vi "Move Impl.vi"(6 "Mode":enum16{"Relative", "Absolute"}(ring), 8 "error in (no error)":errorcluster, 9 "Value (mm)":dbl format="%#_13g", 10 "Axis":T1=enum."Y", 11 "Nikon Ti2 Stage in":refnum<class "Nikon Ti2 Stage.lvclass">) -> (0 "error out":errorcluster, 3 "Nikon Ti2 Stage out":refnum<class "Nikon Ti2 Stage.lvclass">)   [LabVIEW 2023, in "Nikon Ti2 Stage.lvlib" / "Nikon Ti2 Stage.lvclass"]
uses:
  Nikon Ti2 Stage.lvclass
  Stage Controller/Stage Axis.ctl
  Nikon Ti2 Stage.lvclass/Nikon Ti2 Stage.ctl
  Microscope/ti2lv/ti2lv.lvlib
  Stage Controller/Stage Controller.lvclass
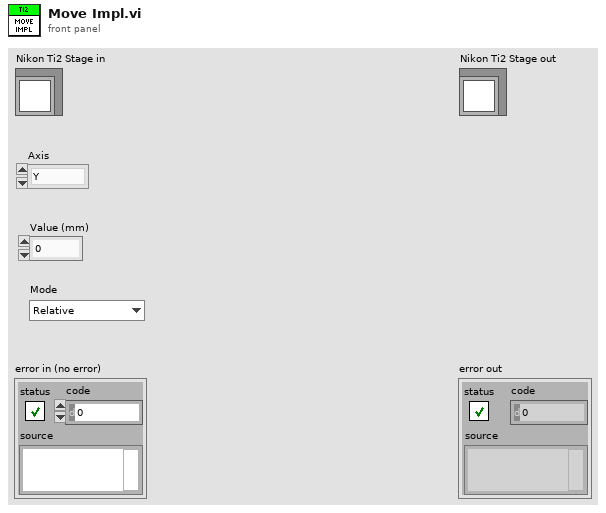
[diagram p1: front panel]
types:
  T1 = typedef "Stage Controller.lvlib/Stage Controller.lvclass/Stage Axis.ctl" = enum16{"unspecified", "X", "Y", "Z"}
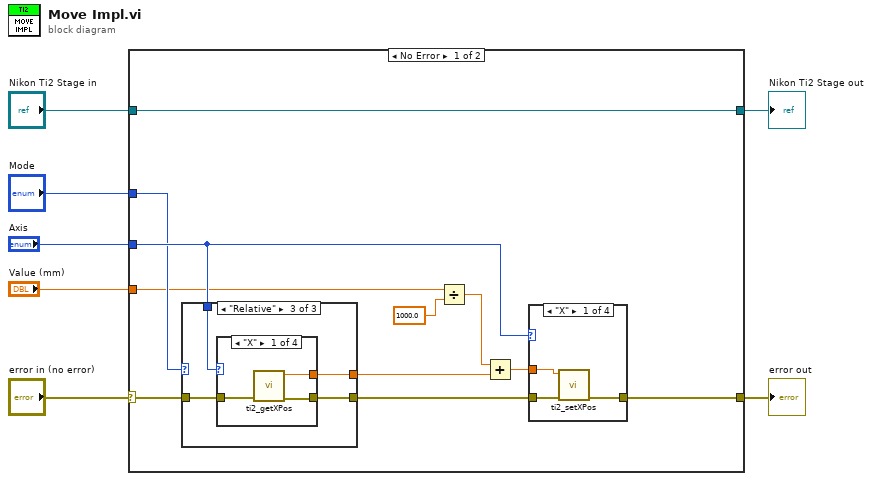
[diagram p0: block diagram]
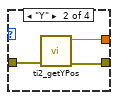
[diagram p4: hidden frame]
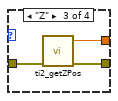
[diagram p5: hidden frame]
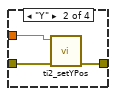
[diagram p7: hidden frame]
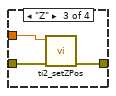
[diagram p8: hidden frame]
diagram:
  n1 = case shown="No Error" "error in (no error)" {
    selector: "error in (no error)" -> [w16 w45]
    tunnel: "Nikon Ti2 Stage in" -> [w18 w46]
    tunnel: [w18 w46] -> w6
    tunnel: [w17 w45] -> w4
    tunnel: "Mode" -> [w13 _]
    tunnel: "Axis" -> [w14 _]
    tunnel: "Value (mm)" -> [w10 _]
    frame No Error {
      n2 = case shown="\"Relative\"" w13 {
        tunnel: w16 -> [w19 w20 w24]
        tunnel: [w19 w20 w23] -> w15
        tunnel: w14 -> [_ _ w22]
        tunnel: [_ _ w21] -> w11
        frame "Absolute" {
        }
        frame Default {
        }
        frame "Relative" {
          n3 = case shown="\"X\"" w22 {
            tunnel: w24 -> [w27 w30 w33 w34]
            tunnel: [w26 w29 w32 w34] -> w23
            tunnel: [w25 w28 w31 _] -> w21
            frame "X" {
              n4 = call "ti2_getXPos.vi"("error in (no error)"=w27) -> ("error out"=w26:errorcluster, "x Position (um)"=w25:dbl)  [unwired: 9 in]
            }
            frame "Y" {
              n5 = call "ti2_getYPos.vi"("error in (no error)"=w30) -> ("error out"=w29:errorcluster, "y Position (um)"=w28:dbl)  [unwired: 9 in]
            }
            frame "Z" {
              n6 = call "ti2_getZPos.vi"("error in (no error)"=w33) -> ("error out"=w32:errorcluster, "z Position (um)"=w31:dbl)  [unwired: 9 in]
            }
            frame Default {
            }
          }
        }
      }
      n7 = Divide(x=w10, y=1000.0) -> (x/y=w9:dbl)
      n8 = Add(x=w9, y=w11) -> (x+y=w12:dbl)
      n9 = case shown="\"X\"" w14 {
        tunnel: w12 -> [w36 w39 w41 _]
        tunnel: [w37 w40 w43 w44] -> w17
        tunnel: w15 -> [w35 w38 w42 w44]
        frame "X" {
          n10 = call "ti2_setXPos.vi"("error in (no error)"=w35, "x Position (um)"=w36) -> ("error out"=w37:errorcluster)  [unwired: 9 in]
        }
        frame "Y" {
          n11 = call "ti2_setYPos.vi"("error in (no error)"=w38, "y Position (um)"=w39) -> ("error out"=w40:errorcluster)  [unwired: 9 in]
        }
        frame "Z" {
          n12 = call "ti2_setZPos.vi"("error in (no error)"=w42, "z Position (um)"=w41) -> ("error out"=w43:errorcluster)  [unwired: 9 in]
        }
        frame Default {
        }
      }
    }
    frame Error {
    }
  }
  "error out" <- w4
  "Nikon Ti2 Stage out" <- w6
